vi "simulate enter button.vi"   [LabVIEW 2021]
uses:
  user32.dll
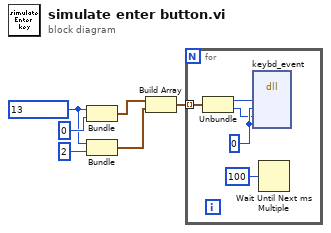
[diagram p0: block diagram]
diagram:
  w2 = u8 13 ("Virtual Key")
  n1 = Bundle("Virtual Key"=w2, 0) -> (w5:cluster{"Virtual Key":u8, i32})  [unwired: 1 in]
  n2 = Bundle("Virtual Key"=w2, 2) -> (w3:cluster{"Virtual Key":u8, i32})  [unwired: 1 in]
  n3 = Build Array(w5, w3) -> (w1:cluster{"Virtual Key":u8, i32}[])
  n4 = for {
    tunnel: w1 -> [w10] mode=indexing
    w11 = u32 0 ("dwFlags")
    n5 = Unbundle(w10) -> ("Virtual Key"=w9:u8, w8:i32)
    n6 = dll-call lib="user32.dll" fn="keybd_event"("bVk"=w9, "bScan"=w11, "dwFlags"=w8, "dwExtraInfo"=w11) -> ()  [unwired: 8 in, 2 out]
    n7 = Wait Until Next ms Multiple(millisecond multiple=u32 100) -> ()  [unwired: 1 out]
  }
